vi "test Loopback Check Status.vi"(8 "error in":errorcluster, 11 "Loopback in":refnum<class "Loopback.lvclass">) -> (0 "error out":errorcluster, 3 "Loopback out":refnum<class "Loopback.lvclass">)   [LabVIEW 2020, in "Loopback.lvclass"]
uses:
  Loopback.lvclass
  C:/dev/git/niveristand-custom-device-testing-tools/VeriStandTestCase/VeriStandTestCase.lvclass
  c61ac340-c88d-49c8-b9fd-f4948625e21f.vi
  <vilib>/NI VeriStand/Execution/Workspace/NI VeriStand - Get Single Channel Value.vi
  <vilib>/NI VeriStand/Execution/Workspace/NI VeriStand - Get Multiple Channel Values.vi
  <vilib>/NI VeriStand/Execution/Workspace/NI_VS Workspace ExecutionAPI.lvlib
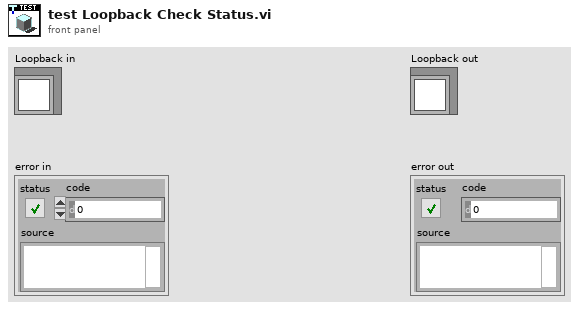
[diagram p1: front panel]
types:
  T1 = typedef "NI_VS Workspace ExecutionAPI.lvlib/WorkspaceAPI.ctl" = refnum<k24>
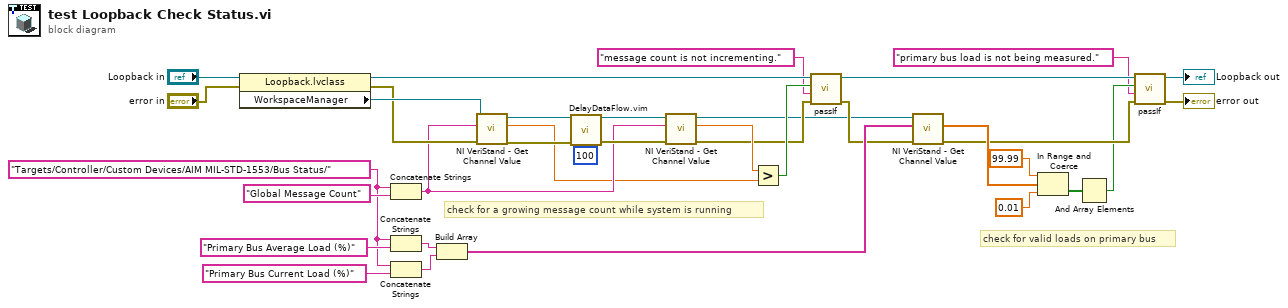
[diagram p0: block diagram]
diagram:
  w17 = "Targets/Controller/Custom Devices/AIM MIL-STD-1553/Bus Status/" ("base name for channel aliases")
  # "check for valid loads on primary bus"
  # "check for a growing message count while system is running"
  n1 = property class="Loopback.lvclass"(reference="Loopback in", error in="error in") -> (reference out=w32:refnum<class "Loopback.lvclass">, error out=w29:errorcluster, "WorkspaceManager"=w30:T1)
  n2 = Concatenate Strings(w17, "Global Message Count" ("base name for channel aliases")) -> (w25:string)
  n3 = Concatenate Strings(w17, "Primary Bus Average Load (%)" ("base name for channel aliases")) -> (w16:string)
  n4 = Concatenate Strings(w17, "Primary Bus Current Load (%)" ("base name for channel aliases")) -> (w15:string)
  n5 = Build Array(w16, w15) -> (w14:string[])
  n6 = call-poly <vilib>:"NI VeriStand - Get Channel Value.vi"("error in (no error)"=w29, "Channel"=w25, "WorkspaceManager in"=w30) -> ("error out"=w28:errorcluster, "Value"=w22:dbl, "WorkspaceManager out"=w24:T1)  [unwired: 6 in]
  n7 = call "DelayDataFlow.vim"("value in"=w28, "milliseconds to wait"=u32 100) -> ("value out"=w26:errorcluster)  [unwired: 2 in, 1 out]
  n8 = call-poly <vilib>:"NI VeriStand - Get Channel Value.vi"("error in (no error)"=w26, "Channel"=w25, "WorkspaceManager in"=w24) -> ("error out"=w20:errorcluster, "Value"=w23:dbl, "WorkspaceManager out"=w12:T1)  [unwired: 6 in]
  n9 = Greater?(x=w23, y=w22) -> (0:w21:bool)
  n10 = call-dynamic "passIf.vi"("error in (no error)"=w20, "message (\"\")"="message count is not incrementing." ("message (\"\")"), "pass"=w21, "TestCase in"=w32) -> ("error out"=w13:errorcluster, "TestCase out"=w4:refnum<class "Loopback.lvclass">)  [unwired: 6 in]
  n11 = call-poly <vilib>:"NI VeriStand - Get Channel Value.vi"("error in (no error)"=w13, "Channels"=w14, "WorkspaceManager in"=w12) -> ("error out"=w7:errorcluster, "Values"=w9:dbl[])  [unwired: 6 in, 1 out]
  n12 = In Range and Coerce(upper limit=99.99, x=w9, lower limit=0.01) -> (In Range?=w8:bool[])  [unwired: 1 out]
  n13 = And Array Elements(Boolean array=w8) -> (logical AND=w6:bool)
  n14 = call-dynamic "passIf.vi"("error in (no error)"=w7, "message (\"\")"="primary bus load is not being measured." ("message (\"\")"), "pass"=w6, "TestCase in"=w4) -> ("error out"=→"error out":errorcluster, "TestCase out"=→"Loopback out":refnum<class "Loopback.lvclass">)  [unwired: 6 in]
